vi "Find Folder in Library.vi"(7 "Library Name":string, 8 "error in (no error)":errorcluster, 9 "Folder Name":string, 10 "Target Name":string, 11 "Project Sync Tools in":refnum<class "Project Sync Tools.lvclass">) -> (0 "error out":errorcluster, 1 "Found?":bool, 2 "Folder Ref out":refnum<vi>, 3 "Project Sync Tools out":refnum<class "Project Sync Tools.lvclass">)   [LabVIEW 2019, in "Project Sync Tools.lvclass"]
uses:
  Project Sync Tools.lvclass
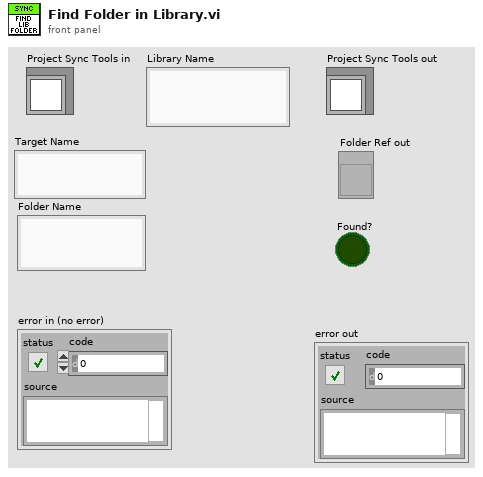
[diagram p1: front panel]
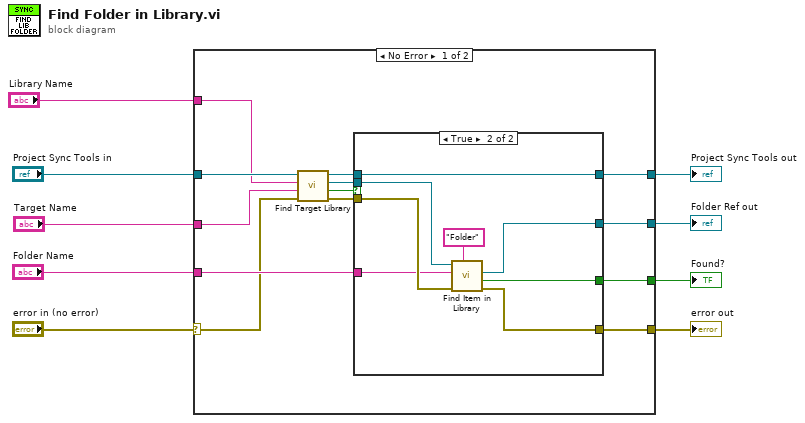
[diagram p0: block diagram]
diagram:
  n1 = case shown="No Error" "error in (no error)" {
    selector: "error in (no error)" -> [w16 w34]
    tunnel: [w22 w34] -> w9
    tunnel: "Folder Name" -> [w21 _]
    tunnel: [w14 w33] -> w7
    tunnel: "Project Sync Tools in" -> [w19 w33]
    tunnel: [w17 _] -> w1
    tunnel: "Target Name" -> [w11 _]
    tunnel: "Library Name" -> [w10 _]
    tunnel: [w12 _] -> w2
    frame No Error {
      n2 = call "Find Target Library.vi"("error in (no error)"=w16, "Target Name"=w11, "Library Name"=w10, "CD Build Tools in"=w19) -> ("error out"=w18:errorcluster, "Found ?"=w15:bool, "Library out"=w20:refnum<vi>, "CD Build Tools out"=w13:refnum<class "Project Sync Tools.lvclass">)  [unwired: 4 in]
      n3 = case shown="True" w15 {
        tunnel: [w24 w32] -> w22
        tunnel: w21 -> [_ w26]
        tunnel: w20 -> [_ w31]
        tunnel: w18 -> [w24 w30]
        tunnel: [_ w29] -> w17
        tunnel: w13 -> [w23 w28]
        tunnel: [w23 w28] -> w14
        tunnel: [_ w25] -> w12
        frame False {
        }
        frame True {
          n4 = call "Find Item in Library.vi"("Type"="Folder", "error in (no error)"=w30, "Item Name"=w26, "Library in"=w31) -> ("error out"=w32:errorcluster, "Found ?"=w25:bool, "ProjectItem out"=w29:refnum<vi>)  [unwired: 4 in, 1 out]
        }
      }
    }
    frame Error {
    }
  }
  "error out" <- w9
  "Project Sync Tools out" <- w7
  "Found?" <- w2
  "Folder Ref out" <- w1
